vi "Generate_Voltage_array_check_size.vi"(4 "output cluster":T1 {"TimeStamp" format="%.2f"}, 5 "error in (no error)":errorcluster, 7 "Number of Steps":i32, 8 "TimeOut Time (s)":dbl format="%.2f") -> (0 "error IO":errorcluster, 1 "DC binary array out":i32[](array[numeric]), 2 "Voltage at each step on PJVS curve 2":dbl[](array[numeric]) format="%#_16g", 3 "Set Frequency":dbl)   [LabVIEW 2020]
uses:
  DataSocketCluster external.ctl
  vi Mode external.ctl
  04bf3837-9317-4129-9531-d6752085829f.vi
  <vilib>/Utility/error.llb/Error Cluster From Error Code.vi
  <vilib>/ErrorRing/Error Ring.xnode
panel:
  out "array":i32[][](array[numeric])
  out "Datasocket return":string
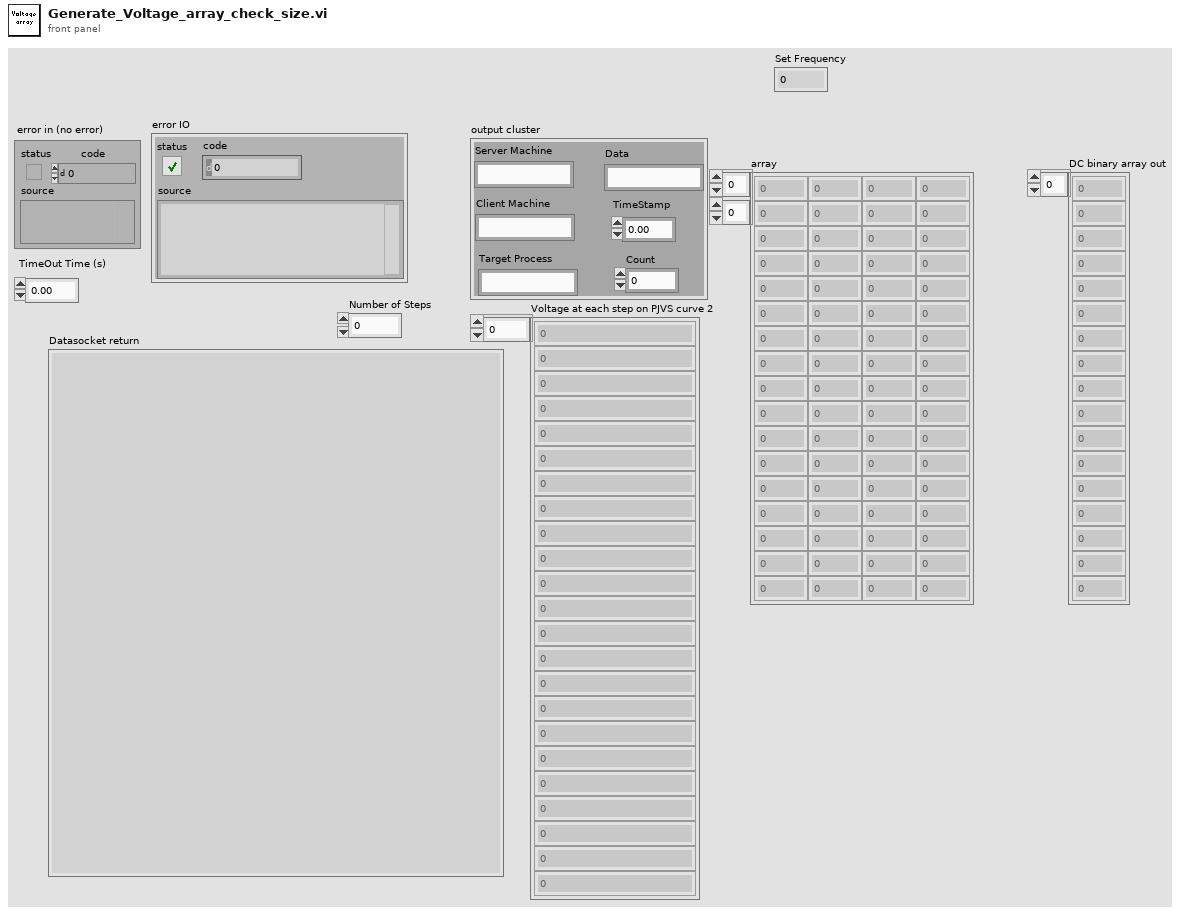
[diagram p1: front panel]
types:
  T1 = typedef "DataSocketCluster external.ctl" = cluster{"Server Machine":string, "Client Machine":string, "Data":string, "TimeStamp":dbl, "Count":i32, "Target Process":string}
  T2 = typedef "vi Mode external.ctl" = enum16{"Client", "Server"}
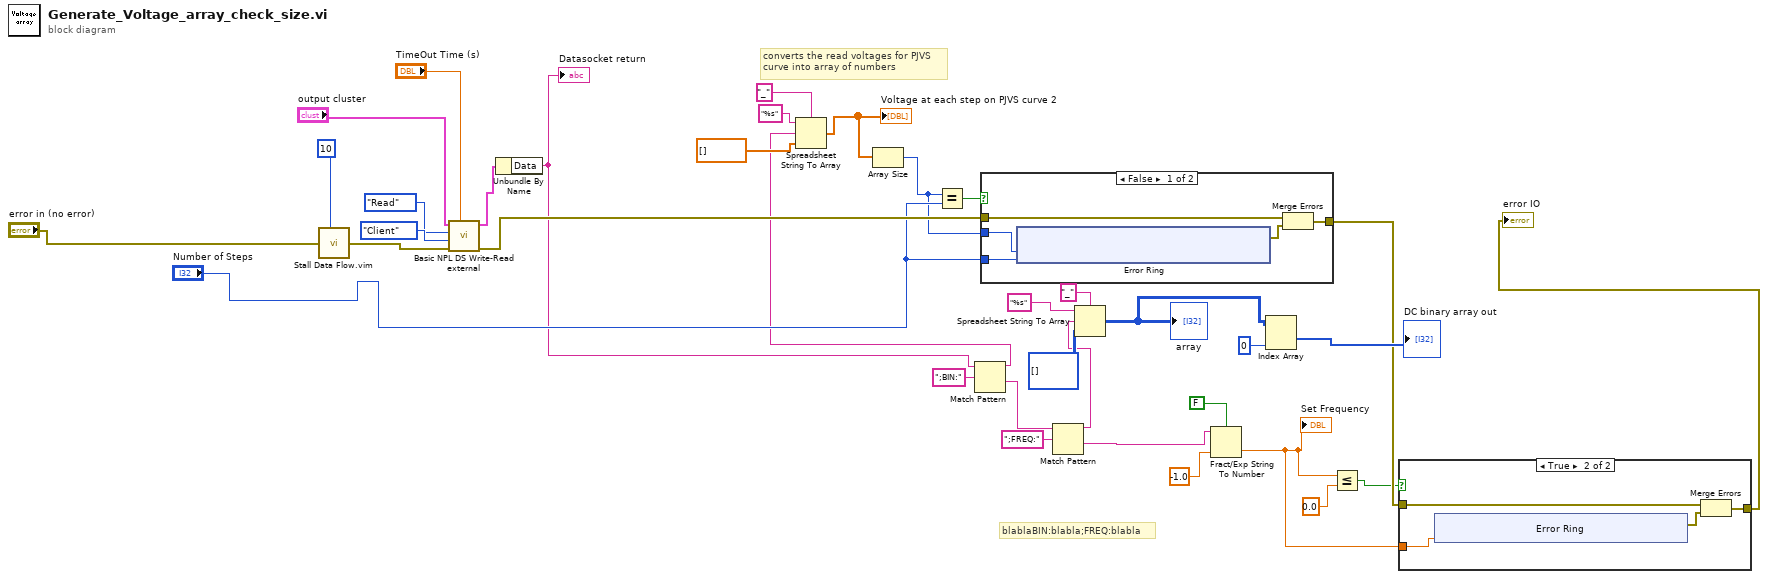
[diagram p0: block diagram]
diagram:
  # "blablaBIN:blabla;FREQ:blabla"
  # "converts the read voltages for PJVS\ncurve into array of numbers"
  n1 = call "Stall Data Flow.vim"("value in"="error in (no error)", "milliseconds to wait"=u32 10) -> ("value out"=w36:errorcluster)  [unwired: 1 out]
  n2 = call "Basic NPL DS Write-Read external.vi"("TimeOut Time (s)"="TimeOut Time (s)", "error in (no error)"=w36, "Server Mode"=vi_Mode_external."Client", "Operation Mode"=enum16{"Read", "Write", "Write/Read"}."Read", "DataSocketCluster In"="output cluster") -> ("error out"=w31:errorcluster, "DataSocketCluster Out"=w30:T1)  [unwired: 2 in, 1 out]
  n3 = Unbundle By Name(w30) -> ("Data"=w18:string)
  "Datasocket return" <- w18
  n4 = Match Pattern(string=w18, regular expression=";BIN:") -> (before substring=w19:string, after substring=w11:string)  [unwired: 1 in, 2 out]
  n5 = Spreadsheet String To Array(delimiter (Tab)="_", format string="%s", spreadsheet string=w19, array type (2D Dbl)=dbl[] []) -> (array=w25:dbl[])
  "Voltage at each step on PJVS curve 2" <- w25
  n6 = Array Size(array=w25) -> (size(s)=w23:i32)
  n7 = Equal?(x=w23, y="Number of Steps") -> (x = y?=w32:bool)
  n8 = case shown="False" w32 {
    tunnel: w31 -> [w38 w50]
    tunnel: w23 -> [w41 _]
    tunnel: "Number of Steps" -> [w40 _]
    tunnel: [w37 w50] -> w5
    frame False {
      n9 = xnode "Error Ring"("parameter 0"=w41, "parameter 1"=w40) -> ("error out"=w39:errorcluster)
      n10 = Merge Errors(w38, w39) -> (w37:errorcluster)
    }
    frame True {
    }
  }
  n11 = Match Pattern(string=w11, regular expression=";FREQ:") -> (before substring=w9:string, after substring=w8:string)  [unwired: 1 in, 2 out]
  n12 = Spreadsheet String To Array(delimiter (Tab)="_" ("format string"), format string="%s", spreadsheet string=w9, array type (2D Dbl)=i32[][] []) -> (array=w14:i32[][])
  "array" <- w14
  n13 = Fract/Exp String To Number(use system decimal point (T)=FALSE, string=w8, default (0 dbl)=-1.0 ("default (0 DBL)")) -> (number=w3:dbl)  [unwired: 1 in, 1 out]
  "Set Frequency" <- w3
  n14 = Index Array(array=w14, index (col)=0 ("index")) -> (element=→"DC binary array out":i32[])  [unwired: 1 in]
  n15 = Less Or Equal?(x=w3, y=0.0) -> (x <= y?=w1:bool)
  n16 = case shown="True" w1 {
    tunnel: w5 -> [w51 w54]
    tunnel: w3 -> [_ w52]
    tunnel: [w51 w53] -> w4
    frame False {
    }
    frame True {
      n17 = xnode "Error Ring"("parameter 0"=w52) -> ("error out"=w55:errorcluster)
      n18 = Merge Errors(w54, w55) -> (w53:errorcluster)
    }
  }
  "error IO" <- w4
